vi "CopyReference.vi"   [LabVIEW 2013]
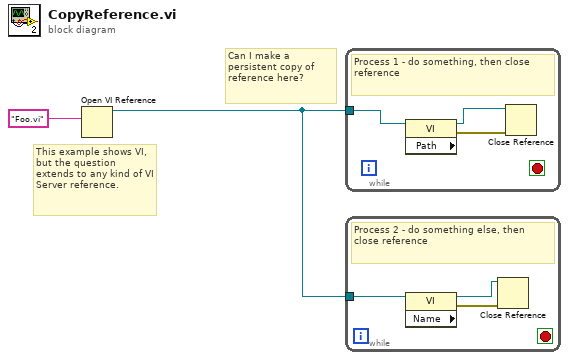
[diagram p0: block diagram]
diagram:
  # "This example shows VI, but the question extends to any kind of VI Server reference."
  # "Can I make a persistent copy of reference here?"
  n1 = Open VI Reference(vi path="Foo.vi") -> (vi reference=w2:refnum<vi>)  [unwired: 5 in, 1 out]
  n2 = while {
    tunnel: w2 -> [w5]
    stop <- _ stop-if-true
    # "Process 1 - do something, then close reference"
    n3 = property class="VI" props=["Path"](reference=w5) -> (reference out=w3:refnum<vi>, error out=w4:errorcluster)  [unwired: 1 in, 1 out]
    n4 = Close Reference(reference=w3, error in (no error)=w4) -> ()  [unwired: 1 out]
  }
  n5 = while {
    tunnel: w2 -> [w8]
    stop <- _ stop-if-true
    # "Process 2 - do something else, then close reference"
    n6 = property class="VI" props=["Name"](reference=w8) -> (reference out=w6:refnum<vi>, error out=w7:errorcluster)  [unwired: 1 in, 1 out]
    n7 = Close Reference(reference=w6, error in (no error)=w7) -> ()  [unwired: 1 out]
  }
